vi "Recieve string from arduino.vi"() -> ()   [LabVIEW 2011]
uses:
  <vilib>/LabVIEW Interface for Arduino/Type Defs/Connection Type.ctl
  <vilib>/LabVIEW Interface for Arduino/Type Defs/Board Type.ctl
  <vilib>/LabVIEW Interface for Arduino/LabVIEW Interface for Arduino.lvlib
panel:
  in  "Tab Control":enum32{"Settings", "Page 2"}(tab)
  in  "Stop Button":bool
  in  "VISA resource name":refnum<visa-resource-name>
  in  "Baud Rate":u32
  in  "Connection Type":T1
  in  "Board Type":T2
  out "Error Out":errorcluster
  in  "size of string sent from arduino":u8
  out "String read from arduino":string
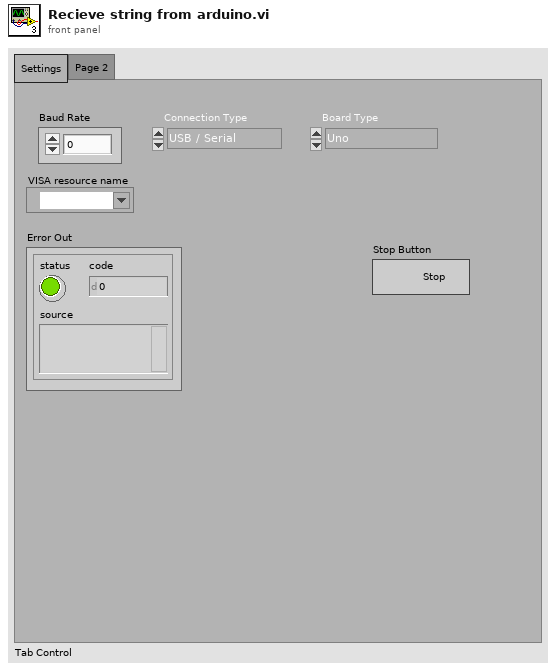
[diagram p1: front panel]
types:
  T1 = typedef "LabVIEW Interface for Arduino.lvlib/Connection Type.ctl" = enum8{"USB / Serial", "XBEE", "BlueSmirf (Bluetooth)"}
  T2 = typedef "LabVIEW Interface for Arduino.lvlib/Board Type.ctl" = enum16{"Uno", "Dimuelanove w/Atmega 328", "Mega 2560"}
  T3 = typedef "LabVIEW Interface for Arduino.lvlib/Arduino Resource.ctl" = cluster{"VISA resource":refnum<visa-resource-name>, "Board Type":T2, "Connection Type":enum8{"USB / Serial"}, "Bytes Per Packet (15)":u8}
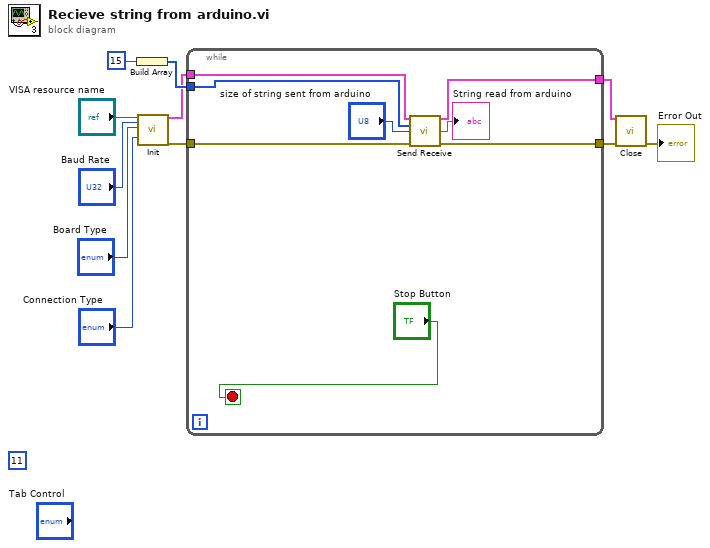
[diagram p0: block diagram]
diagram:
  (unwired) 11
  n1 = Build Array(15) -> (w6:i32[])
  n2 = call <vilib>:"Init.vi"("VISA resource"="VISA resource name", "Baud Rate (115200)"="Baud Rate", "Board Type (Uno)"="Board Type", "Connection Type (USB/Serial)"="Connection Type") -> ("Arduino Resource"=w5:T3, "error out"=w4:errorcluster)  [unwired: 14 in]
  n3 = while {
    tunnel: w6 -> [w18]
    tunnel: w5 -> [w17]
    tunnel: w4 -> [w16]
    tunnel: [w15] -> w1
    tunnel: [w14] -> w3
    stop <- "Stop Button" stop-if-true
    n4 = call <vilib>:"Send Receive.vi"("Arduino Resource"=w17, "Data"=w18, "Bytes To Read (0)"="size of string sent from arduino", "error in"=w16) -> ("Arduino Resource"=w14:T3, "Read Buffer"=→"String read from arduino":string, "error out"=w15:errorcluster)  [unwired: 9 in]
  }
  n5 = call <vilib>:"Close.vi"("Arduino Resource"=w3, "error in"=w1) -> ("error out"=→"Error Out":errorcluster)  [unwired: 13 in]
